vi "test-twist2d.vi"(8 "error in (no error)":errorcluster) -> (0 "error out":errorcluster, 3 "All PASSED":bool)   [LabVIEW 2019]
uses:
  <vilib>/Rock Robotics/WPI/ThirdParty/JAS_Junk/TrajLib/Rotation2d_CreateAngle.vi
  <vilib>/Rock Robotics/WPI/ThirdParty/JAS_Junk/TrajLib/Translation2d_Create.vi
  <vilib>/Rock Robotics/WPI/ThirdParty/JAS_Junk/TrajLib/Trajectory_Library.lvlib
panel:
  out "T3 - Theta - 0":dbl
  out "T3 - X - 0":dbl
  out "T3 - Y - 0":dbl
  out "T2 - Equals - False":bool
  out "T1 - Equals - True":bool
  out "T0 -- Deg -- 0":dbl
  out "T0 -- y -- 0":dbl
  out "T0 -- X -- 0":dbl
  # "Twist2D Test"
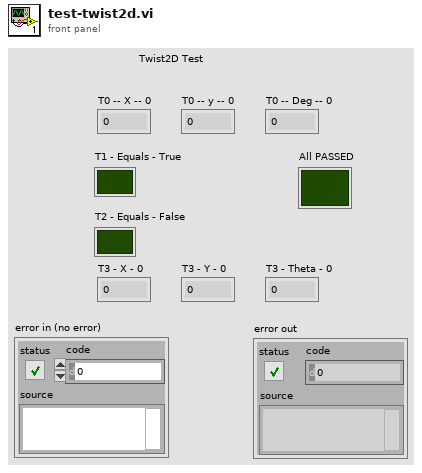
[diagram p1: front panel]
types:
  T1 = typedef "Trajectory_Library.lvlib/POSE2D.ctl" = cluster{"TRANSLATION":T2, "ROTATION":T3}
  T2 = typedef "Trajectory_Library.lvlib/TRANSLATION2D.ctl" = cluster{"X":dbl, "Y":dbl}
  T3 = typedef "Trajectory_Library.lvlib/ROTATION2D.ctl" = cluster{"VALUE":dbl, "COS":dbl, "SIN":dbl}
  T4 = typedef "Trajectory_Library.lvlib/TWIST2D.ctl" = cluster{"dX":dbl, "dY":dbl, "dTHETA":dbl}
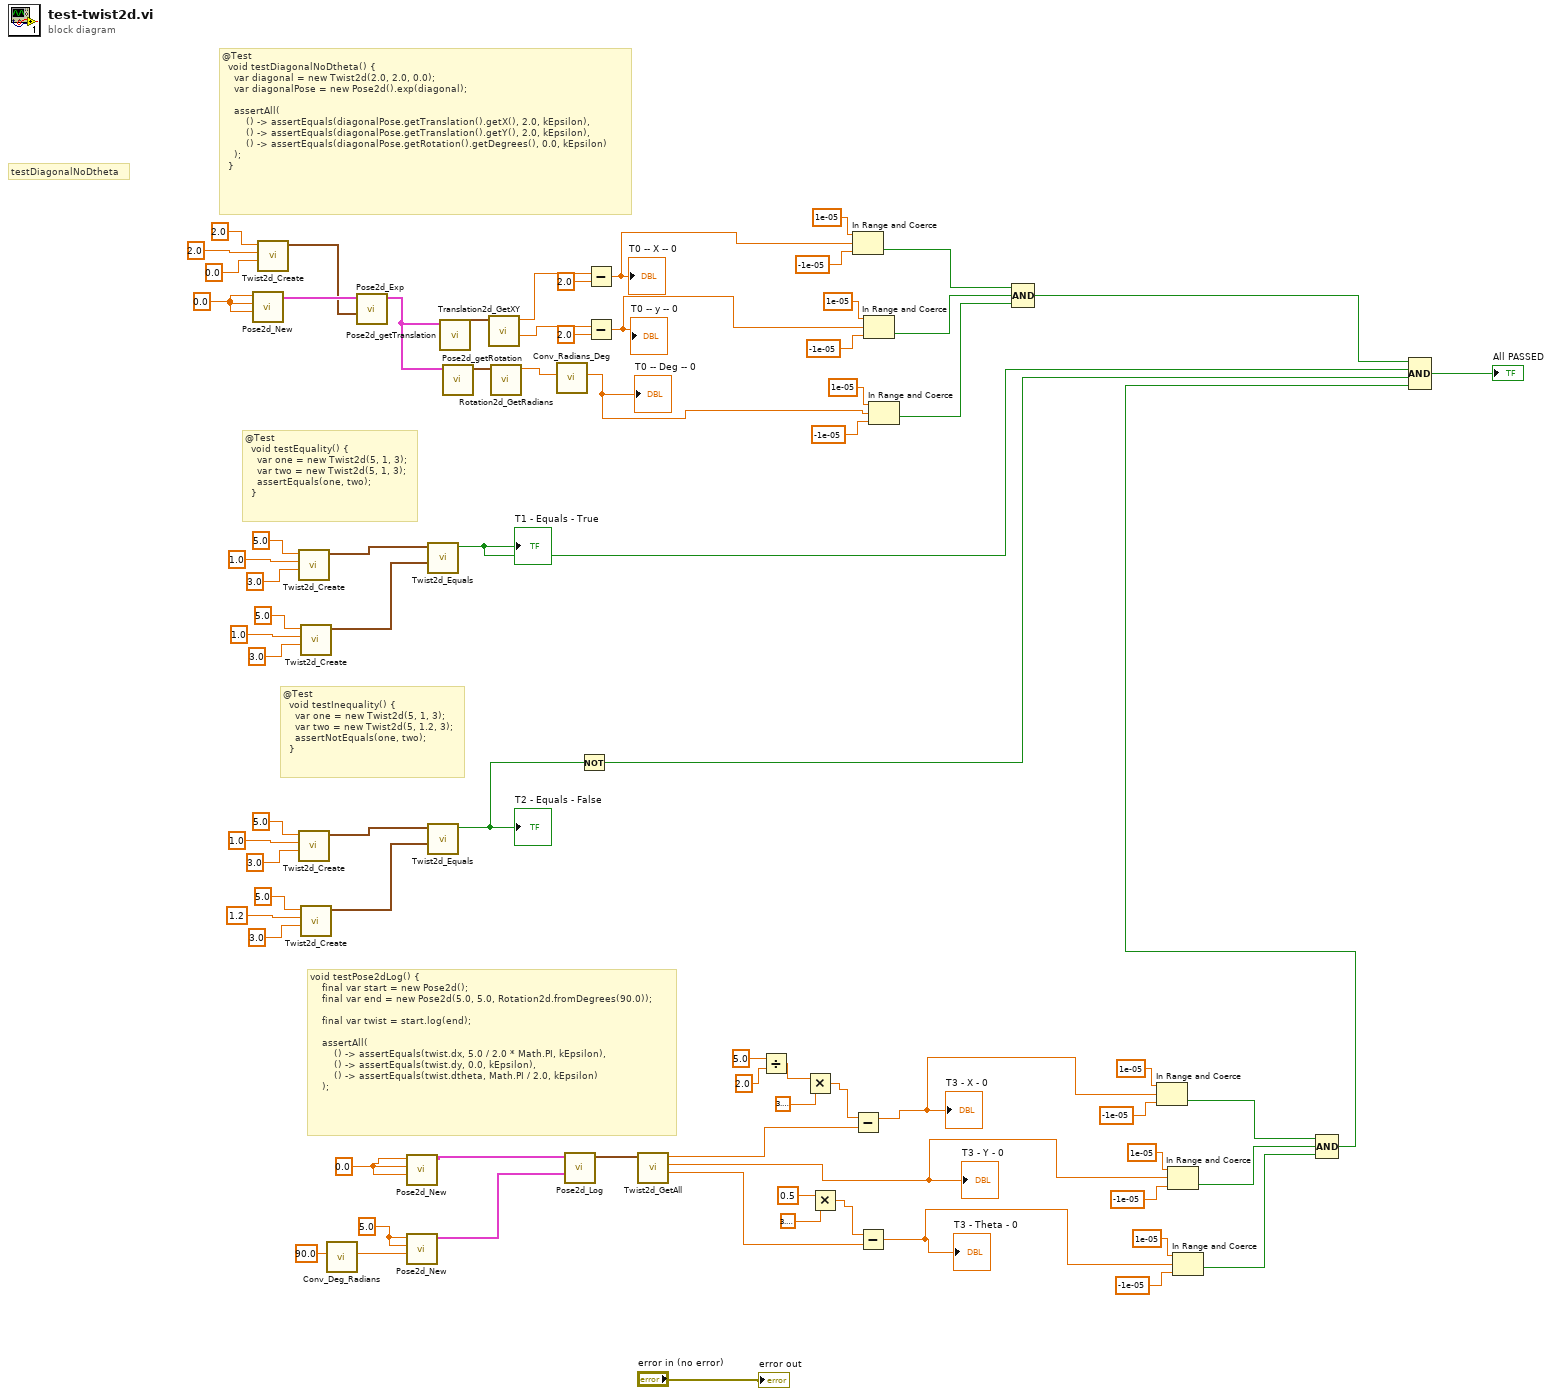
[diagram p0: block diagram]
diagram:
  w47 = 5.0 ("X")
  w32 = 0.0 ("X")
  w75 = 0.0 ("X")
  # "void testPose2dLog() {\n    final var start = new Pose2d();\n    final var end = new Pose2d(5.0, 5.0, Rotation2d.fromDegrees(90.0));\n\n    final var twist = start.log(end);\n\n    assertAll(\n        () -> assertEquals(twist.dx, 5.0 / 2.0 * Math.PI, kEpsilon),\n        () -> assertEquals(twist.dy, 0.0, kEpsilon),\n        () -> assertEquals(twist.dtheta, Math.PI / 2.0, kEpsilon)\n    );"
  # "@Test\n  void testInequality() {\n    var one = new Twist2d(5, 1, 3);\n    var two = new Twist2d(5, 1.2, 3);\n    assertNotEquals(one, two);\n  }"
  # "@Test\n  void testEquality() {\n    var one = new Twist2d(5, 1, 3);\n    var two = new Twist2d(5, 1, 3);\n    assertEquals(one, two);\n  }"
  # "@Test\n  void testDiagonalNoDtheta() {\n    var diagonal = new Twist2d(2.0, 2.0, 0.0);\n    var diagonalPose = new Pose2d().exp(diagonal);\n\n    assertAll(\n        () -> assertEquals(diagonalPose.getTranslation().getX(), 2.0, kEpsilon),\n        () -> assertEquals(diagonalPose.getTranslation().getY(), 2.0, kEpsilon),\n        () -> assertEquals(diagonalPose.getRotation().getDegrees(), 0.0, kEpsilon)\n    );\n  }"
  # "testDiagonalNoDtheta"
  n1 = call <vilib>:"Pose2d_New.vi"("Heading"=w75, "Y"=w75, "X"=w75) -> ("out POSe"=w74:T1)  [unwired: 8 in]
  n2 = call <vilib>:"Twist2d_Create.vi"("dTHETA"=0.0, "dY"=2.0, "dX"=2.0) -> ("TWIST"=w73:T4)  [unwired: 8 in]
  n3 = call <vilib>:"Twist2d_Create.vi"("dTHETA"=3.0, "dY"=1.0, "dX"=5.0) -> ("TWIST"=w58:T4)  [unwired: 8 in]
  n4 = call <vilib>:"Twist2d_Create.vi"("dTHETA"=3.0, "dY"=1.0, "dX"=5.0) -> ("TWIST"=w50:T4)  [unwired: 8 in]
  n5 = call <vilib>:"Twist2d_Create.vi"("dTHETA"=3.0, "dY"=1.0, "dX"=5.0) -> ("TWIST"=w57:T4)  [unwired: 8 in]
  n6 = call <vilib>:"Twist2d_Create.vi"("dTHETA"=3.0, "dY"=1.2, "dX"=5.0) -> ("TWIST"=w49:T4)  [unwired: 8 in]
  n7 = call <vilib>:"Conv_Deg_Radians.vi"("Degress"=90.0) -> ("Radians"=w46:dbl)  [unwired: 10 in]
  n8 = call <vilib>:"Pose2d_Exp.vi"("TWIST"=w73, "POSE"=w74) -> ("UpdatedPose"=w72:T1)  [unwired: 9 in]
  n9 = call <vilib>:"Pose2d_New.vi"("Heading"=w32, "Y"=w32, "X"=w32) -> ("out POSe"=w45:T1)  [unwired: 8 in]
  n10 = call <vilib>:"Pose2d_New.vi"("Heading"=w46, "Y"=w47, "X"=w47) -> ("out POSe"=w44:T1)  [unwired: 8 in]
  n11 = call <vilib>:"Twist2d_Equals.vi"("other TWIST"=w57, "this TWIST"=w58) -> ("Equals"=w4:bool)  [unwired: 9 in]
  "T1 - Equals - True" <- w4
  n12 = call <vilib>:"Twist2d_Equals.vi"("other TWIST"=w49, "this TWIST"=w50) -> ("Equals"=w5:bool)  [unwired: 9 in]
  "T2 - Equals - False" <- w5
  n13 = call <vilib>:"Pose2d_getTranslation.vi"("in POSE"=w72) -> ("outTRANSLATION"=w71:T2)  [unwired: 10 in]
  n14 = call <vilib>:"Pose2d_getRotation.vi"("in POSE"=w72) -> ("out ROTATION"=w70:T3)  [unwired: 10 in]
  n15 = call <vilib>:"Translation2d_GetXY.vi"("In Translation"=w71) -> ("Y"=w66:dbl, "X"=w69:dbl)  [unwired: 9 in]
  n16 = call <vilib>:"Rotation2d_GetRadians.vi"("in ROTATION"=w70) -> ("AngleRadians"=w65:dbl)  [unwired: 10 in]
  n17 = call <vilib>:"Conv_Radians_Deg.vi"("Radians"=w65) -> ("Degrees"=w19:dbl)  [unwired: 10 in]
  "T0 -- Deg -- 0" <- w19
  n18 = call <vilib>:"Pose2d_Log.vi"("end POSE"=w44, "in POSE"=w45) -> ("out TWIST"=w43:T4)  [unwired: 9 in]
  n19 = Not(x=w5) -> (.not. x?=w3:bool)
  n20 = Subtract(x=w69, y=2.0) -> (x-y=w18:dbl)
  "T0 -- X -- 0" <- w18
  n21 = Subtract(x=w66, y=2.0) -> (x-y=w20:dbl)
  "T0 -- y -- 0" <- w20
  n22 = call <vilib>:"Twist2d_GetAll.vi"("TWIST"=w43) -> ("dTHETA"=w33:dbl, "dY"=w7:dbl, "dX"=w37:dbl)  [unwired: 8 in]
  "T3 - Y - 0" <- w7
  n23 = Divide(x=5.0, y=2.0) -> (x/y=w39:dbl)
  n24 = Multiply(x=w39, y=3.141592653589793) -> (x*y=w38:dbl)
  n25 = Multiply(x=0.5, y=3.141592653589793) -> (x*y=w35:dbl)
  n26 = In Range and Coerce(upper limit=1e-05, x=w18, lower limit=-1e-05) -> (In Range?=w26:bool)  [unwired: 1 out]
  n27 = Subtract(x=w38, y=w37) -> (x-y=w8:dbl)
  "T3 - X - 0" <- w8
  n28 = Subtract(x=w35, y=w33) -> (x-y=w6:dbl)
  "T3 - Theta - 0" <- w6
  n29 = In Range and Coerce(upper limit=1e-05, x=w20, lower limit=-1e-05) -> (In Range?=w25:bool)  [unwired: 1 out]
  n30 = In Range and Coerce(upper limit=1e-05, x=w19, lower limit=-1e-05) -> (In Range?=w22:bool)  [unwired: 1 out]
  n31 = Compound Arithmetic op=AND(w26, w25, w22) -> (w21:bool)
  n32 = In Range and Coerce(upper limit=1e-05, x=w8, lower limit=-1e-05) -> (In Range?=w13:bool)  [unwired: 1 out]
  n33 = In Range and Coerce(upper limit=1e-05, x=w7, lower limit=-1e-05) -> (In Range?=w12:bool)  [unwired: 1 out]
  n34 = In Range and Coerce(upper limit=1e-05, x=w6, lower limit=-1e-05) -> (In Range?=w9:bool)  [unwired: 1 out]
  n35 = Compound Arithmetic op=AND(w13, w12, w9) -> (w2:bool)
  n36 = Compound Arithmetic op=AND(w21, w4, w3, w2) -> (→"All PASSED":bool)
  "error out" <- "error in (no error)"
